vi "Find Formula.vi"(8 "error in (no error)":errorcluster, 9 "i in":i32, 11 "VI in":refnum<vi>) -> (0 "error out":errorcluster, 1 "i out":i32, 3 "Array":T1[](array[typedef]))   [LabVIEW 2023, in "VIDoc Parsing.lvlib" / "Structure Reporter.lvlib"]
uses:
  Structure Reporter.lvlib
  Structure Result 2.ctl
  <vilib>/Utility/traverseref.llb/TRef TravTarget.ctl
  <vilib>/Utility/traverseref.llb/VI Scripting - Traverse.lvlib
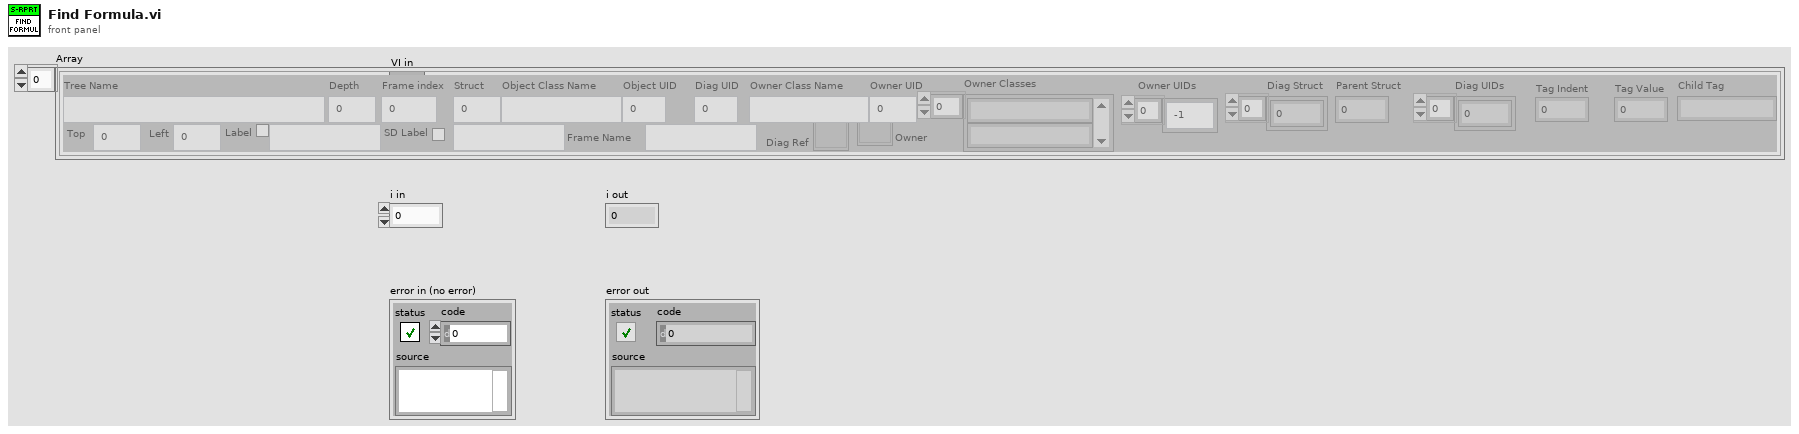
[diagram p1: front panel]
types:
  T1 = typedef "VIDoc Parsing.lvlib/Structure Reporter.lvlib/Structure Result 2.ctl" = cluster{"Depth":i32, "Top":i32, "Left":i32, "Frame index":i32, "Struct":i32, "Object Class Name":string, "Object UID":i32, "Label Visible":bool, "Object Label":string, "SD Label Visible":bool, "Object SD Label":string, "Frame Name":string, "Diag UID":i32, "Owner Class Name":string, "Owner UID":i32, "Diag Struct":i32[], "Parent Struct":i32, "Diag UIDs":i32[], "Tree Name":string, "Diag Ref":refnum<vi>, "Owner Classes":string[], "Owner":refnum<vi>, "Owner UIDs":i32[], "Tag Indent":i32, "Tag Value":i32, "Child Tag":string}
  T2 = typedef "TRef TravTarget.ctl" = enum16{"FP", "BD", "Other"}
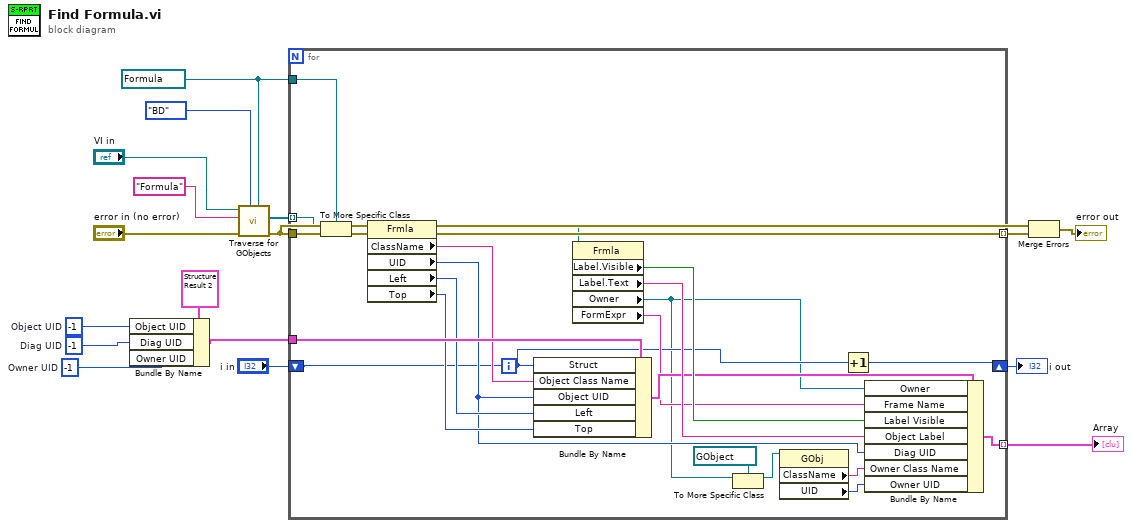
[diagram p0: block diagram]
diagram:
  w3 = -1  # Owner UID
  w4 = -1  # Diag UID
  w5 = -1  # Object UID
  w14 = refnum<vi> refnum ("Other Refnum")
  n1 = Bundle By Name(cluster=T1 {"Depth"=0, "Top"=0, "Left"=0, "Frame index"=0, "Struct"=0, "Object Class Name"="", "Object UID"=0, "Label Visible"=FALSE, "Object Label"="", "SD Label Visible"=FALSE, "Object SD Label"="", "Frame Name"="", "Diag UID"=0, "Owner Class Name"="", "Owner UID"=0, "Diag Struct"=[], "Parent Struct"=0, "Diag UIDs"=[], "Tree Name"="", "Diag Ref"=refnum, "Owner Classes"=[], "Owner"=refnum, "Owner UIDs"=[], "Tag Indent"=0, "Tag Value"=0, "Child Tag"=""}, "Object UID"=w5, "Diag UID"=w4, "Owner UID"=w3) -> (w2:T1)
  n2 = call <vilib>:"Traverse for GObjects.vi"("Other Refnum"=w14, "Traverse Target"=TRef_TravTarget."BD", "error in (no error)"="error in (no error)", "Class Name"="Formula", "VI Refnum"="VI in") -> ("error out"=w1:errorcluster, "References"=w15:refnum<vi>[])  [unwired: 3 in, 2 out]
  n3 = for {
    tunnel: w15 -> [w39] mode=indexing
    tunnel: w14 -> [w38]
    tunnel: w2 -> [w37]
    tunnel: [w25] -> w16 mode=indexing
    tunnel: w1 -> [w23]
    tunnel: [w22] -> w10 mode=indexing
    shift-right: [w19] -> w7
    shift-left: "i in" -> [w20]
    n4 = To More Specific Class(target class=w38, reference=w39, error in=w23) -> (specific class reference=w40:refnum<vi>, error out=w41:errorcluster)
    n5 = property class="Frmla"(reference=w40, error in=w41) -> (reference out=w21:refnum<vi>, error out=w22:errorcluster, "ClassName"=w36:string, "UID"=w24:i32, "Left"=w35:i32, "Top"=w34:i32)
    n6 = Bundle By Name(cluster=w37, "Struct"=w20, "Object Class Name"=w36, "Object UID"=w24, "Left"=w35, "Top"=w34) -> (w27:T1)
    n7 = property class="Frmla"(reference=w21) -> ("Label.Visible"=w33:bool, "Label.Text"=w28:string, "Owner"=w18:refnum<vi>, "FormExpr"=w26:string)  [unwired: 1 in, 2 out]
    n8 = To More Specific Class(target class=refnum<vi> refnum ("Other Refnum"), reference=w18) -> (specific class reference=w31:refnum<vi>)  [unwired: 1 in, 1 out]
    n9 = property class="GObj"(reference=w31) -> ("ClassName"=w30:string, "UID"=w29:i32)  [unwired: 1 in, 2 out]
    n10 = Increment(x=w20) -> (x+1=w19:i32)
    n11 = Bundle By Name(cluster=w27, "Owner"=w18, "Frame Name"=w26, "Label Visible"=w33, "Object Label"=w28, "Diag UID"=w24, "Owner Class Name"=w30, "Owner UID"=w29) -> (w25:T1)
  }
  "Array" <- w16
  "i out" <- w7
  n12 = Merge Errors(w1, w10) -> (→"error out":errorcluster)
